vi "HTTP GET.vi"(6 "request specific headers":T1[](array[typedef]), 8 "error in (no error)":errorcluster, 10 "Path":string, 11 "REST Client in":refnum<class "REST Client.lvclass">) -> (0 "error out":errorcluster, 1 "Response body":string, 2 "Response Headers":refnum<class "Response Headers.lvclass">, 3 "REST Client out":refnum<class "REST Client.lvclass">, 4 "Status String":string, 5 "Status Code":u16)   [LabVIEW 2013, in "REST Client.lvlib" / "REST Client.lvclass"]
doc: "Perform a HTTP GET request.\n\nThe VI provides multiple arguments for defining how to perform the HTTP request.\n\n<b>Path</b> specifies the path beneath the Base URL to be used for the HTTP request.\nrequest specific headers specifies an array of headers to be used with this particular HTTP request. \n\n<b>request specific headers</b> The Default Headers specified upon creation of the JKI REST Client together with the request specific headers will all be used for the HTTP request."
uses:
  REST Client.lvclass
  Response Headers/Response Headers.lvclass
  HTTP Header.ctl
  HTTP Methods.ctl
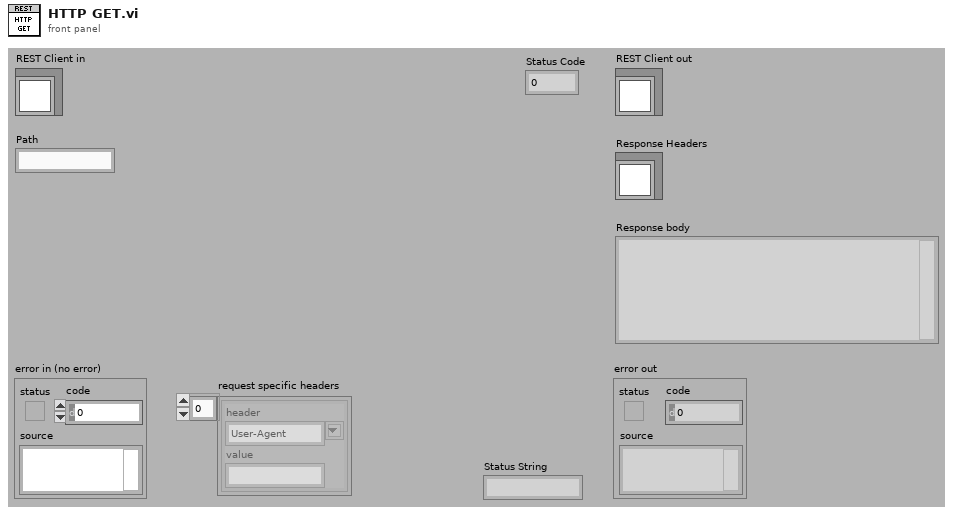
[diagram p1: front panel]
types:
  T1 = typedef "REST Client.lvlib/REST Client.lvclass/HTTP Header.ctl" = cluster{"header":string, "value":string}
  T2 = typedef "REST Client.lvlib/REST Client.lvclass/HTTP Methods.ctl" = enum16{"GET", "HEAD", "POST", "PUT", "DELETE"}
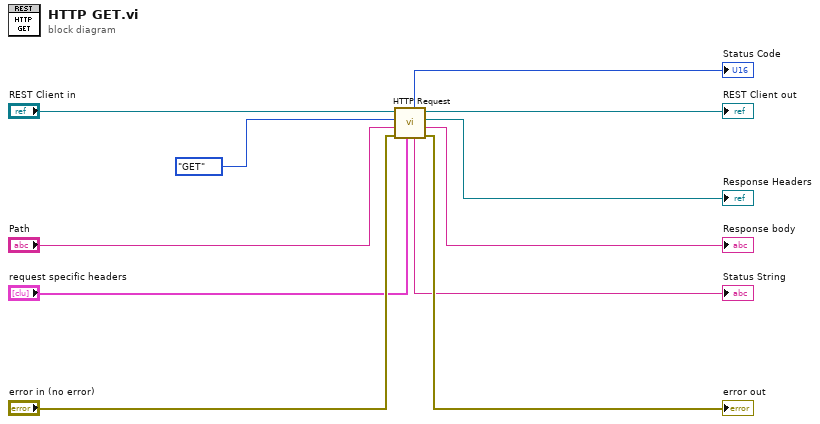
[diagram p0: block diagram]
diagram:
  n1 = call-dynamic "HTTP Request.vi"("request specific headers"="request specific headers", "error in (no error)"="error in (no error)", "Path"="Path", "Method"=HTTP_Methods."GET", "REST Client in"="REST Client in") -> ("error out"=→"error out":errorcluster, "Response body"=→"Response body":string, "Response Headers out"=→"Response Headers":refnum<class "Response Headers.lvclass">, "REST Client out"=→"REST Client out":refnum<class "REST Client.lvclass">, "Status String"=→"Status String":string, "Status Code"=→"Status Code":u16)  [unwired: 1 in]
